vi "Communication Initialized.vi"(8 "error in (no error)":errorcluster, 9 "com_port":refnum<visa-resource-name>, 10 "com_source":T1(ring)) -> (0 "error out":errorcluster)   [LabVIEW 2018, in "1039_mod.lvlib"]
doc: "_____\nCreated using Delacor QMH Event Scripter 4.2.1.88."
uses:
  1039_mod.lvlib
  Initialize Communication Argument--cluster.ctl
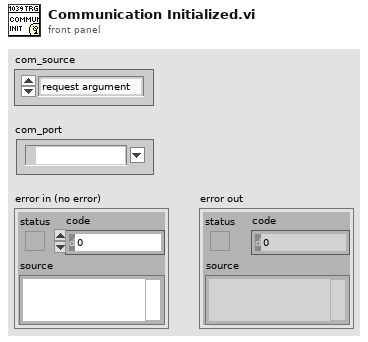
[diagram p1: front panel]
types:
  T1 = enum16{"request argument", "configuration file", "module setting"}
  T2 = typedef "1039_mod.lvlib/Initialize Communication Argument--cluster.ctl" = cluster{"com_source":enum16{"request argument", "configuration file", "module setting"}, "com_port":refnum<visa-resource-name>}
  T3 = typedef "1039_mod.lvlib/Broadcast Events--cluster.ctl" = cluster{"Module Did Init":refnum<user-event>, "Status Updated":refnum<user-event>, "Error Reported":refnum<user-event>, "Module Did Stop":refnum<user-event>, "Update Module Execution Status":refnum<user-event>, "Communication Initialized":refnum<user-event>, "Instrument Initialized":refnum<user-event>, "Instrument Configured":refnum<user-event>}
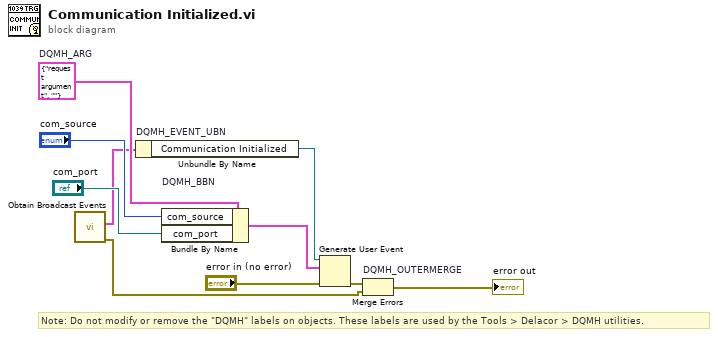
[diagram p0: block diagram]
diagram:
  w5 = T2 {"com_source"=enum."request argument", "com_port"=""}  # DQMH_ARG
  # "Note: Do not modify or remove the \"DQMH\" labels on objects. These labels are used by the Tools > Delacor > DQMH utilities."
  n1 = call "Obtain Broadcast Events.vi"() -> ("error out"=w2:errorcluster, "1039_mod Broadcast Events"=w1:T3)  [unwired: 10 in]
  n2 = Unbundle By Name "DQMH_EVENT_UBN"(w1) -> ("Communication Initialized"=w7:refnum<user-event>)
  n3 = Bundle By Name "DQMH_BBN"(cluster=w5, "com_source"="com_source", "com_port"="com_port") -> (w8:T2)
  n4 = Generate User Event(user event=w7, event data cluster=w8, error in="error in (no error)") -> (error out=w6:errorcluster)  [unwired: 1 in, 1 out]
  n5 = Merge Errors "DQMH_OUTERMERGE"(w6, w2) -> (→"error out":errorcluster)
